vi "WaveformAcquisitionSynchronous.vi"() -> ()   [LabVIEW 2012]
uses:
  <vilib>/Utility/file.llb/Read From Spreadsheet File (DBL).vi
  <vilib>/Utility/file.llb/Write To Spreadsheet File (DBL).vi
  Madlib.dll
panel:
  in  "Axis":u32
  in  "Number of Steps":u32=2 min=2 max=1000
  in  "DAC Rate (ms)":dbl=1.0 min=0.0333333 max=5.0 format="%.4f"
  in  "Write Waveform To":path
  in  "Load Waveform From":path
  in  "ADC Rate (ms)":dbl=1.0 min=0.033333 max=5.0 format="%.4f"
  in  "Number of Positions to Read":u32=2 min=2 max=1000
  out "Waveform Graph":dbl[](graph)
  # "This example demonstrates the two step process of simultaneous triggering a waveform read/write on a single axis.\nPosition control data (separated by spaces) is loaded from a specified basic text file (Load Waveform From) and \nposition data read from the axis is appended to a file (Write Waveform To)."
  # "X = 1\nY = 2\nZ = 3"
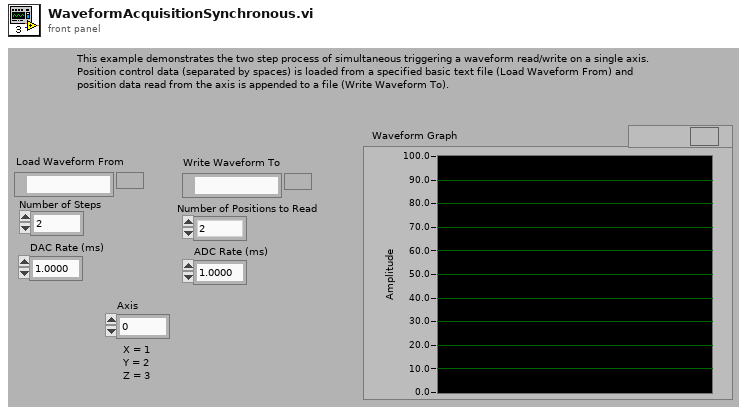
[diagram p1: front panel]
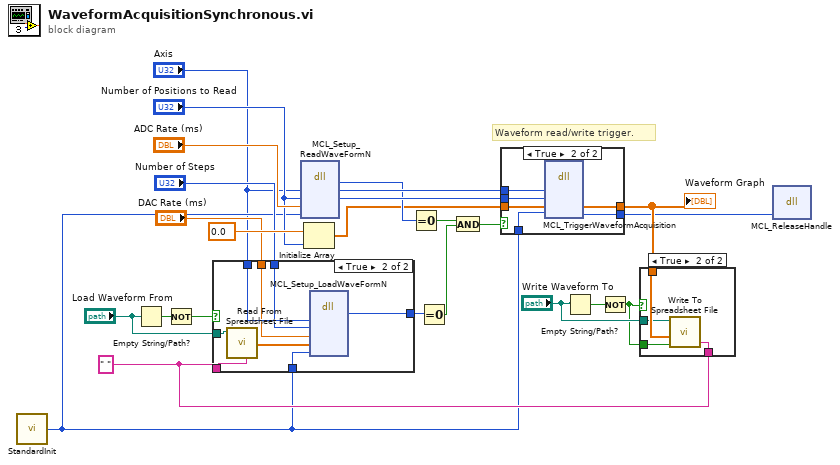
[diagram p0: block diagram]
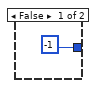
[diagram p3: hidden frame]
diagram:
  w4 = " "
  # "Waveform read/write trigger."
  n1 = call "StandardInit.vi"() -> ("Outgoing Handle"=w2:i32)  [unwired: 1 in]
  n2 = Empty String/Path?(string/path="Load Waveform From") -> (empty?=w15:bool)
  n3 = Not(x=w15) -> (.not. x?=w14:bool)
  n4 = case shown="True" w14 {
    tunnel: [-1 w33] -> w18
    tunnel: "Axis" -> [_ w32]
    tunnel: "Load Waveform From" -> [_ w31]
    tunnel: "DAC Rate (ms)" -> [_ w30]
    tunnel: "Number of Steps" -> [_ w28]
    tunnel: w4 -> [_ w27]
    tunnel: w2 -> [_ w26]
    frame False {
    }
    frame True {
      n5 = call-poly <vilib>:"Read From Spreadsheet File.vi"("delimiter (\\t)"=w27, "file path (dialog if empty)"=w31) -> ("first row"=w29:dbl[])  [unwired: 5 in, 4 out]
      n6 = dll-call lib="C:/Users/Labview/Desktop/SRR/Madlib_x64/Labview Examples/MADLib.dll" fn="MCL_Setup_LoadWaveFormN" label="Setup WF Load"("axis"=w32, "DataPoints"=w28, "milliseconds"=w30, "waveform"=w29, "handle"=w26) -> (w33:i32)  [unwired: 8 in, 2 out]
    }
  }
  n7 = dll-call lib="C:/Users/Labview/Desktop/SRR/Madlib_x64/Labview Examples/MADLib.dll" fn="MCL_Setup_ReadWaveFormN" label="Setup WF Read"("axis"="Axis", "DataPoints"="Number of Positions to Read", "milliseconds"="ADC Rate (ms)", "handle"=w2) -> (w19:i32, "axis"=w22:u32, "DataPoints"=w21:u32)  [unwired: 5 in, 2 out]
  n8 = Initialize Array(0.0, "Number of Positions to Read") -> (w7:dbl[])
  n9 = Equal To 0?(x=w19) -> (x = 0?=w24:bool)
  n10 = Equal To 0?(x=w18) -> (x = 0?=w23:bool)
  n11 = And(x=w24, y=w23) -> (x .and. y?=w20:bool)
  n12 = case shown="True" w20 {
    tunnel: [_ w40] -> w10
    tunnel: w22 -> [_ w39]
    tunnel: w21 -> [_ w38]
    tunnel: w7 -> [_ w37]
    tunnel: w2 -> [w34 w36]
    tunnel: [w34 w35] -> w3
    frame False {
    }
    frame True {
      n13 = dll-call lib="C:/Users/Labview/Desktop/SRR/Madlib_x64/Labview Examples/MADLib.dll" fn="MCL_TriggerWaveformAcquisition"("axis"=w39, "DataPoints"=w38, "waveform"=w37, "handle"=w36) -> ("waveform"=w40:dbl[], "handle"=w35:i32)  [unwired: 6 in, 2 out]
    }
  }
  "Waveform Graph" <- w10
  n14 = Empty String/Path?(string/path="Write Waveform To") -> (empty?=w13:bool)
  n15 = Not(x=w13) -> (.not. x?=w11:bool)
  n16 = case shown="True" w11 {
    tunnel: w10 -> [_ w44]
    tunnel: "Write Waveform To" -> [_ w43]
    tunnel: w11 -> [_ w42]
    tunnel: w4 -> [_ w41]
    frame False {
    }
    frame True {
      n17 = call-poly <vilib>:"Write To Spreadsheet File.vi"("delimiter (\\t)"=w41, "append to file? (new file:F)"=w42, "1D data"=w44, "file path (dialog if empty)"=w43) -> ()  [unwired: 4 in, 1 out]
    }
  }
  n18 = dll-call lib="C:/Users/Labview/Desktop/SRR/Madlib_x64/Labview Examples/MADLib.dll" fn="MCL_ReleaseHandle"("handle"=w3) -> ()  [unwired: 5 in, 2 out]
